vi "Cs++Actor exist.vi"(8 "Error In":errorcluster, 11 "Actor Name":string) -> (0 "Error Out":errorcluster, 2 "Exist?":bool, 3 "dup Actor Name":string)   [LabVIEW 2015, in "CS++Utilities.lvlib"]
doc: "Check if the specified actor was already launched."
uses:
  CS++Utilities.lvlib
  Base/FGV Action.ctl
  Base/CS++Base.lvlib
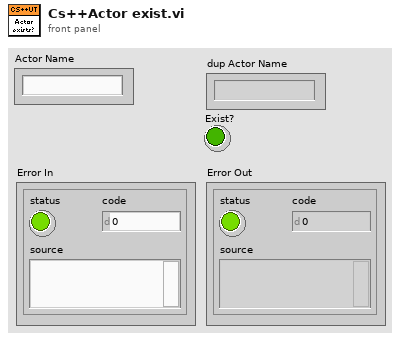
[diagram p1: front panel]
types:
  T1 = typedef "CS++Base.lvlib/FGV Action.ctl" = enum16{"add", "replace", "read", "remove", "reset", "get attributes"}
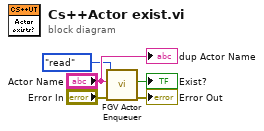
[diagram p0: block diagram]
diagram:
  n1 = call "FGV Actor Enqueuer.vi"("Error In"="Error In", "Actor Name"="Actor Name", "Action (read)"=FGV_Action."read") -> ("Error Out"=→"Error Out":errorcluster, "Success"=→"Exist?":bool)  [unwired: 4 in, 3 out]
  "dup Actor Name" <- "Actor Name"
